vi "createCsvFile.vi"(8 "error in (no error)":errorcluster, 10 "data\\fileName.csv":string, 11 "Header 1, Header 2, etc.":string) -> (0 "error out":errorcluster, 3 "Byte Stream File out":refnum<file>)   [LabVIEW 2019]
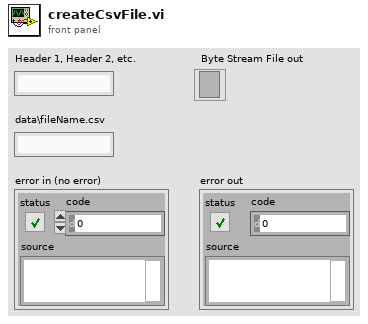
[diagram p1: front panel]
types:
  T1 = enum32{"invalid app kind", "Development System", "Run Time System", "Student Edition", "Embedded LabVIEW", "Evaluation", "Custom"}
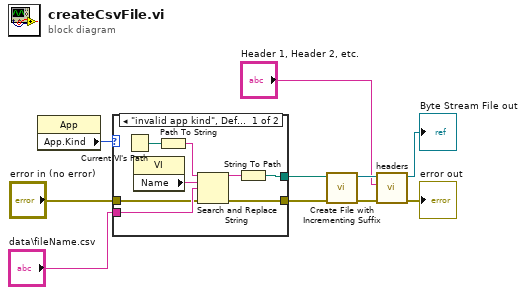
[diagram p0: block diagram]
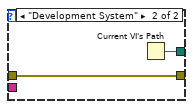
[diagram p2: hidden frame]
diagram:
  n1 = property class="App"() -> ("App.Kind"=w5:T1)  [unwired: 2 in, 2 out]
  n2 = case shown="\"invalid app kind\", Default" w5 {
    tunnel: [w18 w20] -> w4
    tunnel: "data\\fileName.csv" -> [w13 _]
    tunnel: [w12 w19] -> w6
    tunnel: "error in (no error)" -> [w11 w19]
    frame "invalid app kind", Default {
      n3 = Current VI's Path() -> (path=w15:path)
      n4 = property class="VI"() -> ("Name"=w14:string)  [unwired: 2 in, 2 out]
      n5 = Path To String(path=w15) -> (string=w16:string)
      n6 = Search and Replace String(input string=w16, search string=w14, replace string=w13, error in=w11) -> (result string=w17:string, error out=w12:errorcluster)  [unwired: 4 in, 2 out]
      n7 = String To Path(string=w17) -> (path=w18:path)
    }
    frame "Development System" {
      n8 = Current VI's Path() -> (path=w20:path)
    }
  }
  n9 = call <vilib>:"Create File with Incrementing Suffix.vi"("error in (no error)"=w6, "file path"=w4) -> ("error out"=w8:errorcluster, "refnum out"=w7:refnum<file>)  [unwired: 7 in, 1 out]
  n10 = call "headers.vi"("error in (no error)"=w8, "string"="Header 1, Header 2, etc.", "Byte Stream File in"=w7) -> ("error out"=→"error out":errorcluster, "Byte Stream File out"=→"Byte Stream File out":refnum<file>)  [unwired: 7 in]
